vi "PRIME Detector Update FITS Header offsets.vi"() -> ()   [LabVIEW 2024, in "PRIME Detector.lvclass"]
uses:
  PRIME Detector.lvclass
  RIMAS Detector Config.ctl
  RIMAS Detector Server Config.ctl
  RIMAS Observation Config.ctl
  Detector enum Detector Integration Mode.ctl
  Detector Image typedef cluster.ctl
  Detector Class.lvclass
panel:
  out "Error out":errorcluster
  in  "Error in":errorcluster
  in  "Images":T1[](array[typedef])
  in  "Detector Config":T2={"Detector"=0, "Offsets"=[[0, 0, 0, 0, 0, 0, 0, 0, 0, 0, 0, 0, 0, 0, 0, 0, 0, 0, 0, 0, 0, 0, 0, 0, 0, 0, 0, 0, 0, 0, 0, 0]], "Detector Computer"={"Machine"="192.168.121.11", "Password"="", "FITS File Path"="", "Port"=44444, "Header Path"="", "Name"=""}, "FITS hdr template0"=path "", "FITS hdr template1"=path "", "FITS Data File Path"=path "", "FITS Detector Settings"={"Exp Time Short"=0.0, "# of Frames"=0.0, "Exp Time Long"=0.0, "# of Groups"=0.0, "Object Name"="", "Object"="", "Obs Type"="", "Image Type"="", "Observer"="", "Observer Affiliation"=""}, "Sim Folder"=path "", "Integration Mode"=enum."Ramp", "Integration Time"=0.0, "Frame Int Time"=0.0} {"Offsets" format="%04x"; "Detector" items=["0", "1", "2"]}
  # "sec"
  # "sec"
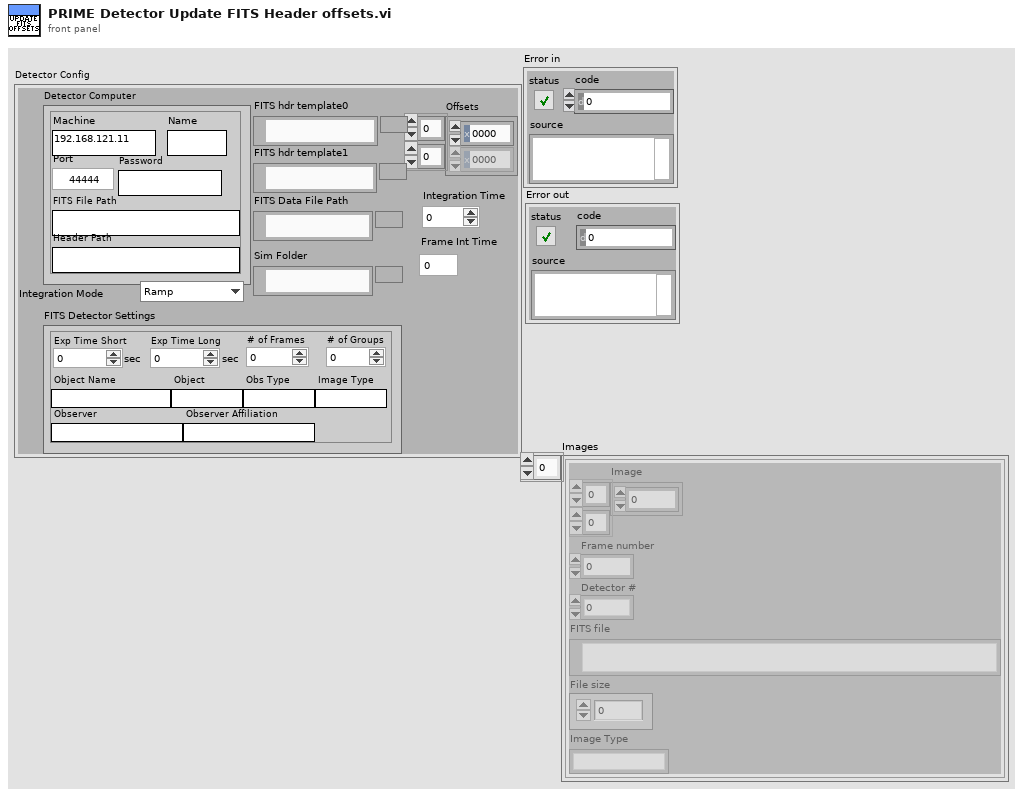
[diagram p1: front panel]
types:
  T1 = typedef "Detector Class.lvclass/Detector Image typedef cluster.ctl" = cluster{"Image":sgl[][], "Frame number":i32, "Detector #":u16, "FITS file":path, "File size":i64, "Image Type":string}
  T2 = typedef "RIMAS Detector Config.ctl" = cluster{"Detector":u16, "Offsets":u16[][], "Detector Computer":T3, "FITS hdr template0":path, "FITS hdr template1":path, "FITS Data File Path":path, "FITS Detector Settings":T4, "Sim Folder":path, "Integration Mode":T5, "Integration Time":dbl, "Frame Int Time":dbl}
  T3 = typedef "RIMAS Detector Server Config.ctl" = cluster{"Machine":string, "Password":string, "FITS File Path":string, "Port":u16, "Header Path":string, "Name":string}
  T4 = typedef "RIMAS Observation Config.ctl" = cluster{"Exp Time Short":dbl, "# of Frames":dbl, "Exp Time Long":dbl, "# of Groups":dbl, "Object Name":string, "Object":string, "Obs Type":string, "Image Type":string, "Observer":string, "Observer Affiliation":string}
  T5 = typedef "Detector enum Detector Integration Mode.ctl" = enum16{"Ramp", "CDS", "FOWLER2", "FOWLER4", "FOWLER8", "FOWLER16", "Raw"}
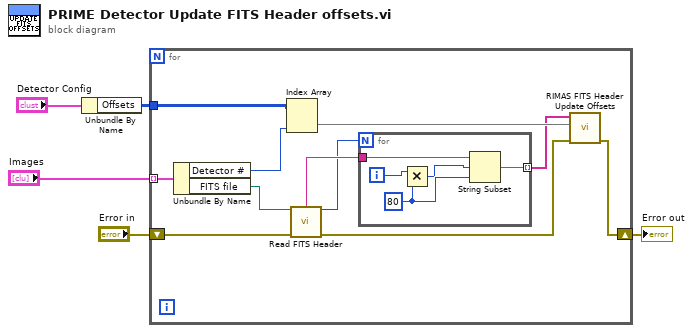
[diagram p0: block diagram]
diagram:
  n1 = Unbundle By Name("Detector Config") -> ("Offsets"=w3:u16[][])
  n2 = for {
    tunnel: "Images" -> [w16] mode=indexing
    tunnel: w3 -> [w15]
    shift-right: [w8] -> w1
    shift-left: "Error in" -> [w12]
    n3 = Unbundle By Name(w16) -> ("Detector #"=w11:u16, "FITS file"=w13:path)
    n4 = Index Array(array=w15, index (col)=w11) -> (element=w14:u16[])  [unwired: 1 in]
    n5 = call "Read FITS Header.vi"("Input File:"=w13, "error in"=w12) -> ("Header"=w10:string, "Header Lines"=w9:i32, "error out"=w6:errorcluster)  [unwired: 4 in, 7 out]
    n6 = for {
      N: w9 -> [_]
      tunnel: w10 -> [w21]
      tunnel: [w17] -> w7 mode=indexing
      i -> [w19]
      w20 = 80 ("length (rest)")
      n7 = Multiply(x=w19, y=w20) -> (x*y=w18:i32)
      n8 = String Subset(string=w21, offset (0)=w18, length (rest)=w20) -> (substring=w17:string)
    }
    n9 = call "RIMAS FITS Header Update Offsets.vi"("Error In"=w6, "Offsets"=w14, "header file"=w7) -> ("Error Out"=w8:errorcluster)  [unwired: 7 in, 1 out]
  }
  "Error out" <- w1
